vi "zlgcan_demo_I.vi"() -> ()   [LabVIEW 2018]
uses:
  data_type/ZCAN_InitCAN_setting_I.ctl
panel:
  in  "工作模式":u8(ring) items=["正常", "只听"]
  in  "屏蔽码":u32=4294967295 format="%x"
  in  "验收码":u32
  in  "滤波模式":u8(ring) items=["双滤波", "单滤波"]
  in  "自定义波特率字符输入":string
  in  "使用自定义波特率？":bool
  in  "波特率":u32(ring)=500000 items=["1Mbps"=1000000, "800kbps"=800000, "500kbps"=500000, "250kbps"=250000, "125kbps"=125000, "100kbps"=100000, "50kbps"=50000]
  in  "通道索引":u32(ring) items=["0", "1", "2", "3"]
  in  "设备索引":u32(ring) items=["0", "1", "2", "3"]
  in  "设备类型":u32(ring)=4 items=["PCI-9810"=2, "USBCAN-II"=4, "USBCAN-E-U"=20, "USBCANFD-100U"=42, "USBCANFD-200U"=41, "PCIE-CANFD-100U"=38, "PCIE-CANFD-200U"=39, "PCIE-CANFD-400U"=40, "云设备"=46]
  in  "开启CAN":bool
  in  "stop":bool
  in  "ID":u32 format="0x%08x"
  in  "数据长度(最大8字节)":u8=8 max=8
  in  "Data Byte 8":u8 caption="data88" format="%.0x"
  in  "Data Byte 7":u8 caption="data7" format="%.0x"
  in  "Data Byte 6":u8 caption="data6" format="%.0x"
  in  "Data Byte 5":u8 caption="data5" format="%.0x"
  in  "Data Byte 4":u8 caption="data4" format="%.0x"
  in  "Data Byte 3":u8 caption="data3" format="%.0x"
  in  "Data Byte 2":u8 caption="data2" format="%.0x"
  in  "Data Byte 1":u8 caption="data1" format="%.0x"
  in  "帧格式":u32(ring) items=["数据帧", "远程帧"]
  in  "发送方式":u32(ring) items=["正常发送", "单次发送", "自发自收", "单次自发自收"]
  in  "帧类型":u32(ring) items=["标准帧", "扩展帧"]
  in  "每次发送帧数":u32=1
  in  "发送":bool
  out "can_index_handle(out)":u32
  out "Device_handle(out)":u32
  in  "I系列初始化参数":T1
  out "已接收帧数":u32
  out "接收字符串显示":string caption="String"
  # "停止程序前，需要先关闭CAN卡"
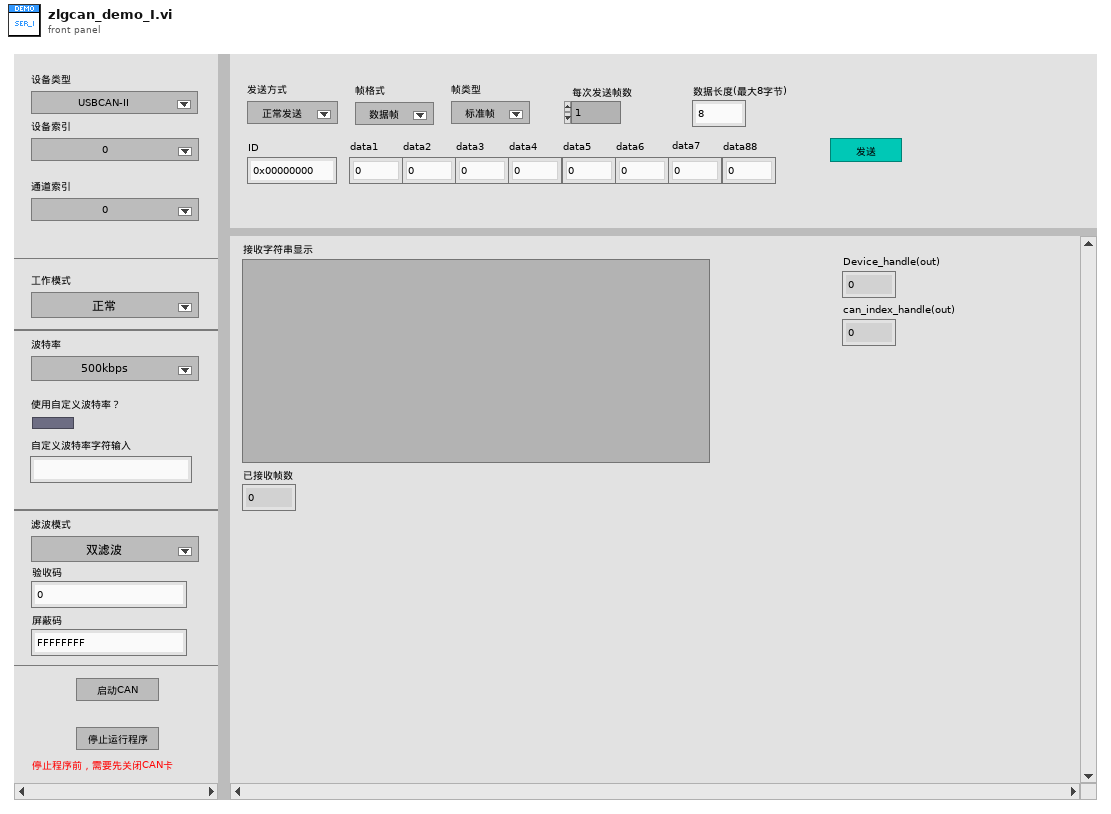
[diagram p1: front panel]
types:
  T1 = typedef "ZCAN_InitCAN_setting_I.ctl" = cluster{"baudrate":u32, "baud_rate_custom？":bool, "RateCustom":string, "filter":u8, "acc_code":u32, "acc_mask":u32, "mode":u8}
  T2 = cluster{"[0]":u8, "[1]":u8, "[2]":u8, "[3]":u8, "[4]":u8, "[5]":u8, "[6]":u8, "[7]":u8}
  T3 = cluster{u32, u8, u8, u8, u8, cluster{"[0]":u8, "[1]":u8, "[2]":u8, "[3]":u8, "[4]":u8, "[5]":u8, "[6]":u8, "[7]":u8}, u64}[]
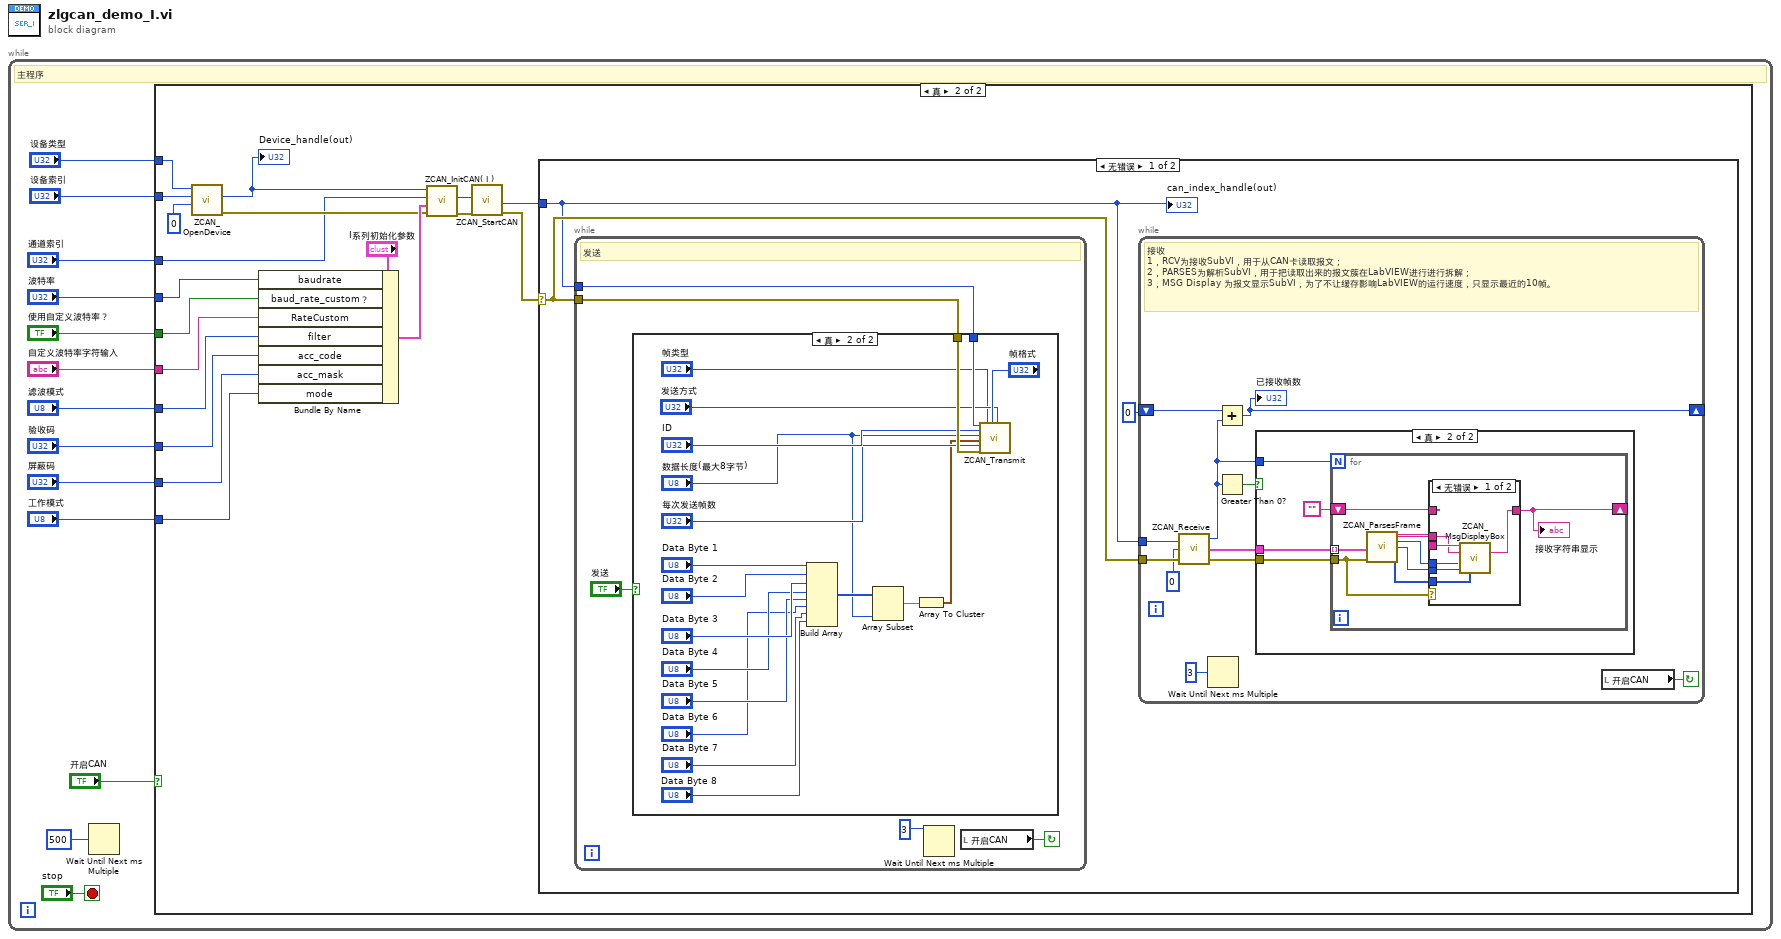
[diagram p0: block diagram]
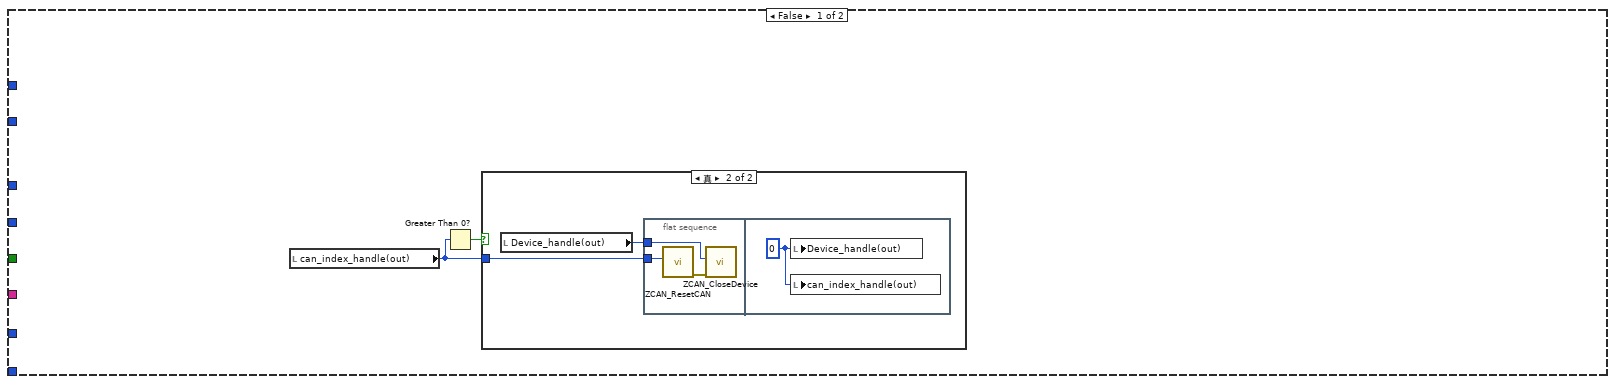
[diagram p2: hidden frame]
diagram:
  n1 = while {
    stop <- "stop" stop-if-true
    # "主程序"
    n2 = Wait Until Next ms Multiple(millisecond multiple=u32 500) -> ()  [unwired: 1 out]
    n3 = case shown="真" "开启CAN" {
      tunnel: "通道索引" -> [_ w22]
      tunnel: "波特率" -> [_ w30]
      tunnel: "使用自定义波特率？" -> [_ w29]
      tunnel: "自定义波特率字符输入" -> [_ w36]
      tunnel: "工作模式" -> [_ w33]
      tunnel: "验收码" -> [_ w35]
      tunnel: "屏蔽码" -> [_ w34]
      tunnel: "设备类型" -> [_ w31]
      tunnel: "设备索引" -> [_ w32]
      tunnel: "滤波模式" -> [_ w28]
      frame False {
        # "关闭CAN卡"
        n4 = local read "can_index_handle(out)"() -> (w14:u32)
        n5 = Greater Than 0?(x=w14) -> (x > 0?=w15:bool)
        n6 = case shown="真" w15 {
          tunnel: w14 -> [_ w17]
          frame False {
          }
          frame True {
            n7 = local read "Device_handle(out)"() -> (w16:u32)
            n8 = flat-sequence {
              tunnel: w17 -> [w19]
              tunnel: w16 -> [w18]
              frame #0 {
                n9 = call "ZCAN_ResetCAN.vi"("can_handle"=w19) -> ("error out"=w20:errorcluster)  [unwired: 9 in, 1 out]
                n10 = call "ZCAN_CloseDevice.vi"("error in (no error)"=w20, "device_handle"=w18) -> ()  [unwired: 8 in, 2 out]
              }
              frame #1 {
                w21 = u32 0 ("can_index_handle(out)")
                n11 = local write "Device_handle(out)"(w21) -> ()
                n12 = local write "can_index_handle(out)"(w21) -> ()
              }
            }
          }
        }
      }
      frame True {
        n13 = call "ZCAN_OpenDevice.vi"("reserved"=0, "device_index"=w32, "device_type"=w31) -> ("error out"=w26:errorcluster, "DEVICE_HANDLE"=w23:u32)  [unwired: 7 in]
        "Device_handle(out)" <- w23
        n14 = Bundle By Name(cluster="I系列初始化参数", "baudrate"=w30, "baud_rate_custom？"=w29, "RateCustom"=w36, "filter"=w28, "acc_code"=w35, "acc_mask"=w34, "mode"=w33) -> (w37:T1)
        n15 = call "ZCAN_InitCAN( I ).vi"("error in (no error)"=w26, "I系列初始化参数"=w37, "can_index"=w22, "device_hande"=w23) -> ("error out"=w39:errorcluster, "can_index_handle"=w38:u32)  [unwired: 2 in]
        n16 = call "ZCAN_StartCAN.vi"("error in (no error)"=w39, "can_index_handle"=w38) -> ("error out"=w24:errorcluster, "can_index_handle(out)"=w25:u32)  [unwired: 7 in, 1 out]
        n17 = case shown="无错误" w24 {
          selector: w24 -> [w42 _]
          tunnel: w25 -> [w41 _]
          frame No Error {
            n18 = while {
              tunnel: w41 -> [w77]
              tunnel: w42 -> [w75]
              stop <- w76 continue-if-true
              # "发送"
              n19 = case shown="真" "发送" {
                tunnel: w77 -> [_ w98]
                tunnel: w75 -> [_ w97]
                frame False {
                }
                frame True {
                  n20 = Build Array("Data Byte 1", "Data Byte 2", "Data Byte 3", "Data Byte 4", "Data Byte 5", "Data Byte 6", "Data Byte 7", "Data Byte 8") -> (w84:u8[])
                  n21 = Array Subset(array=w84, length="数据长度(最大8字节)") -> (w82:u8[])  [unwired: 1 in]
                  n22 = Array To Cluster(array=w82) -> (cluster=w81:T2)
                  n23 = call "ZCAN_Transmit.vi"("can_index_handle"=w98, "ID"="ID", "数据长度"="数据长度(最大8字节)", "DATA"=w81, "每次发送帧数"="每次发送帧数", "error in (no error)"=w97, "帧类型"="帧类型", "帧格式"="帧格式", "发送方式"="发送方式") -> ()  [unwired: 10 in, 1 out]
                }
              }
              n24 = Wait Until Next ms Multiple(millisecond multiple=u32 3) -> ()  [unwired: 1 out]
              n25 = local read "开启CAN"() -> (w76:bool)
            }
            n26 = while {
              tunnel: w42 -> [w51]
              tunnel: w41 -> [w49]
              shift-right: [w52] -> _
              shift-left: 0 -> [w53]
              stop <- w44 continue-if-true
              # "接收\n1，RCV为接收SubVI，用于从CAN卡读取报文；\n2，PARSES为解析SubVI，用于把读取出来的报文簇在LabVIEW进行进行拆解；\n3，MSG Display 为报文显示SubVI，为了不让缓存影响LabVIEW的运行速度，只显示最近的10帧。"
              n27 = call "ZCAN_Receive.vi"("error in (no error)"=w51, "type"=u8 0, "can_handle"=w49) -> ("error out"=w47:errorcluster, "Receive"=w48:T3, "Receive_Num"=w46:u32)
              n28 = Wait Until Next ms Multiple(millisecond multiple=u32 3) -> ()  [unwired: 1 out]
              n29 = Add(x=w53, y=w46) -> (x+y=w52:u32)
              "已接收帧数" <- w52
              n30 = Greater Than 0?(x=w46) -> (x > 0?=w45:bool)
              n31 = case shown="真" w45 {
                tunnel: w46 -> [_ w58]
                tunnel: w48 -> [_ w57]
                tunnel: w47 -> [_ w56]
                frame False {
                }
                frame True {
                  n32 = for {
                    N: w58 -> [_]
                    tunnel: w57 -> [w65] mode=indexing
                    tunnel: w56 -> [w64]
                    shift-right: [w67] -> _
                    shift-left: "" -> [w66]
                    n33 = call "ZCAN_ParsesFrame.vi"("ZCAN_Receive_Data"=w65, "error in (no error)"=w64) -> ("帧格式"=w59:string, "帧类型"=w60:string, "ID"=w61:u32, "data_len"=w63:u8, "data"=w62:u8[])  [unwired: 8 in, 1 out]
                    n34 = case shown="无错误" w64 {
                      tunnel: [w73 w74] -> w67
                      tunnel: w66 -> [_ w74]
                      tunnel: w63 -> [w72 _]
                      tunnel: w62 -> [w71 _]
                      tunnel: w61 -> [w70 _]
                      tunnel: w60 -> [w69 _]
                      tunnel: w59 -> [w68 _]
                      frame No Error {
                        n35 = call "ZCAN_MsgDisplayBox.vi"("帧类型"=w69, "ID"=w70, "帧格式"=w68, "Message Data"=w71, "data_len"=w72) -> ("Output String"=w73:string)  [unwired: 10 in]
                      }
                      frame Error {
                      }
                    }
                    "接收字符串显示" <- w67
                  }
                }
              }
              n36 = local read "开启CAN"() -> (w44:bool)
            }
            "can_index_handle(out)" <- w41
          }
          frame Error {
          }
        }
      }
    }
  }
